vi "结果转换成字符串数组.vi"(10 "结果数据数组簇":T1) -> (2 "结果字符串数组簇":T2)   [LabVIEW 2020]
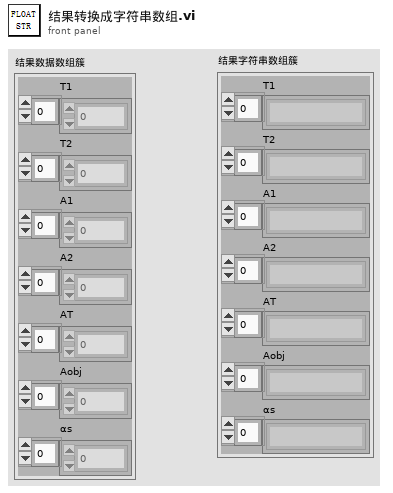
[diagram p1: front panel]
types:
  T1 = cluster{"T1":dbl[], "T2":dbl[], "A1":dbl[], "A2":dbl[], "AT":dbl[], "Aobj":dbl[], "αs":dbl[]}
  T2 = cluster{"T1":string[], "T2":string[], "A1":string[], "A2":string[], "AT":string[], "Aobj":string[], "αs":string[]}
  T3 = cluster{string[], string[], string[], string[], string[], string[], string[]}
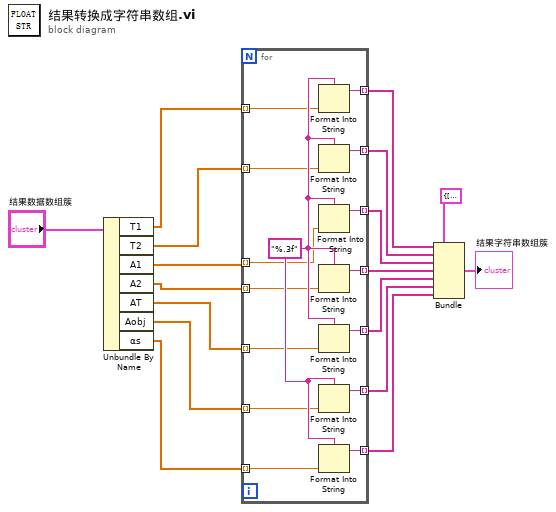
[diagram p0: block diagram]
diagram:
  n1 = Unbundle By Name("结果数据数组簇") -> ("T1"=w7:dbl[], "T2"=w6:dbl[], "A1"=w5:dbl[], "A2"=w4:dbl[], "AT"=w3:dbl[], "Aobj"=w2:dbl[], "αs"=w1:dbl[])
  n2 = for {
    tunnel: [w32] -> w11 mode=indexing
    tunnel: [w31] -> w15 mode=indexing
    tunnel: [w30] -> w14 mode=indexing
    tunnel: [w29] -> w13 mode=indexing
    tunnel: [w28] -> w12 mode=indexing
    tunnel: [w26] -> w16 mode=indexing
    tunnel: [w25] -> w17 mode=indexing
    tunnel: w7 -> [w24] mode=indexing
    tunnel: w6 -> [w23] mode=indexing
    tunnel: w5 -> [w22] mode=indexing
    tunnel: w4 -> [w21] mode=indexing
    tunnel: w3 -> [w20] mode=indexing
    tunnel: w2 -> [w19] mode=indexing
    tunnel: w1 -> [w18] mode=indexing
    w27 = "%.3f" ("格式字符串")
    n3 = Format Into String(format string=w27, w24) -> (resulting string=w25:string)  [unwired: 2 in, 1 out]
    n4 = Format Into String(format string=w27, w23) -> (resulting string=w26:string)  [unwired: 2 in, 1 out]
    n5 = Format Into String(format string=w27, w22) -> (resulting string=w31:string)  [unwired: 2 in, 1 out]
    n6 = Format Into String(format string=w27, w21) -> (resulting string=w30:string)  [unwired: 2 in, 1 out]
    n7 = Format Into String(format string=w27, w20) -> (resulting string=w29:string)  [unwired: 2 in, 1 out]
    n8 = Format Into String(format string=w27, w19) -> (resulting string=w28:string)  [unwired: 2 in, 1 out]
    n9 = Format Into String(format string=w27, w18) -> (resulting string=w32:string)  [unwired: 2 in, 1 out]
  }
  n10 = Bundle(cluster=T3 {[], [], [], [], [], [], []} ("簇"), w17, w16, w15, w14, w13, w12, w11) -> (→"结果字符串数组簇":T3)
